vi "LabView Motor Controller.vi"() -> ()   [LabVIEW 2025]
uses:
  <vilib>/Instr/_visa.llb/VISA Configure Serial Port (Instr).vi
panel:
  in  "Start Looping Sequence":bool
  in  "Loop: Distance To Travel":dbl
  in  "Loop: Number of Cycles":dbl
  out "Current Status":string
  in  "RESET":bool
  in  "Zero":bool
  in  "Speed":dbl
  in  "Go To Location":dbl
  in  "Move Steps":dbl
  in  "VISA resource name":refnum<visa-resource-name>
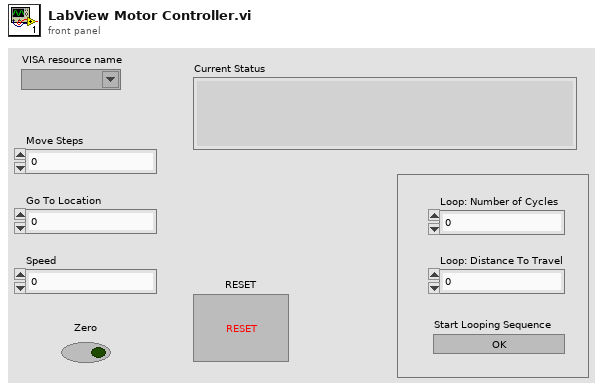
[diagram p1: front panel]
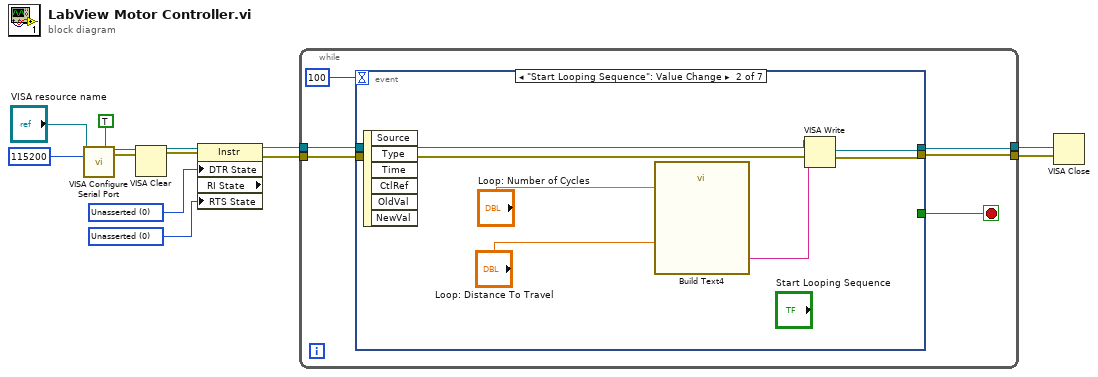
[diagram p0: block diagram]
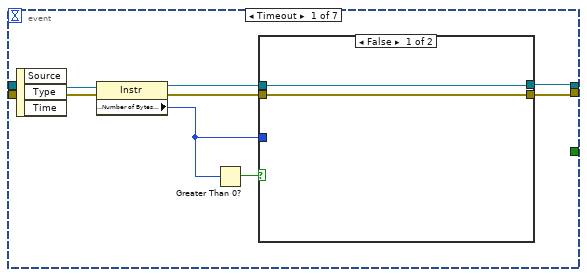
[diagram p2: hidden frame]
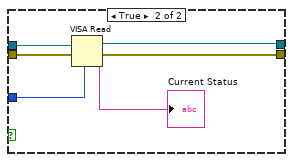
[diagram p3: hidden frame]
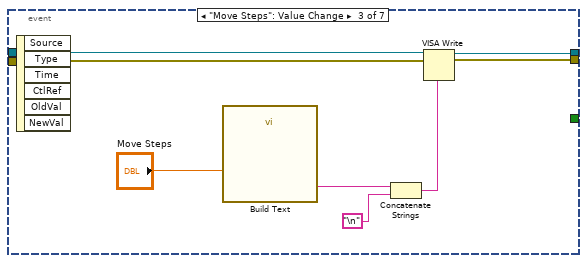
[diagram p4: hidden frame]
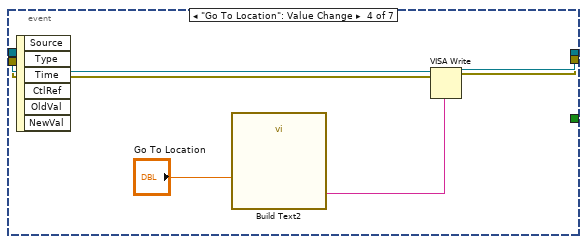
[diagram p5: hidden frame]
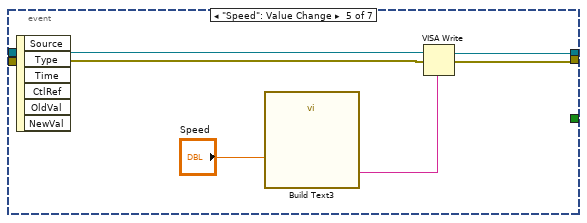
[diagram p6: hidden frame]
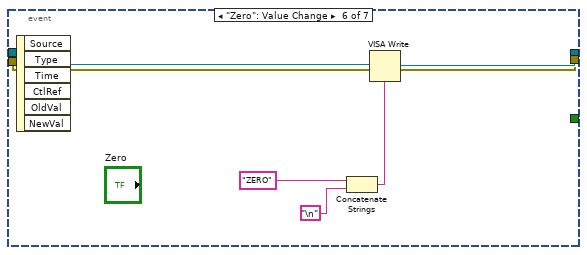
[diagram p7: hidden frame]
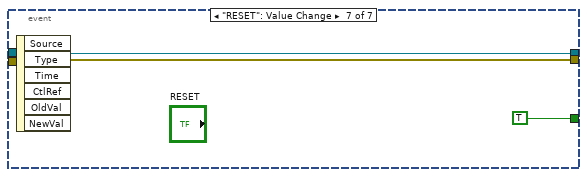
[diagram p8: hidden frame]
diagram:
  w5 = i16 0 items=["Unknown"=-1, "Unasserted"=0, "Asserted"=1] ("Serial Settings:Modem Line Settings:Line DTR State")
  w6 = i16 0 items=["Unknown"=-1, "Unasserted"=0, "Asserted"=1] ("Serial Settings:Modem Line Settings:Line RTS State")
  n1 = call-poly "VISA Configure Serial Port"("VISA resource name"="VISA resource name", "Enable Termination\nChar (T)"=TRUE ("Enable Termination\nChar (T)"), "baud rate (9600)"=u32 115200) -> ("VISA resource name out"=w4:refnum<visa-resource-name>, "error out"=w3:errorcluster)  [unwired: 11 in]
  n2 = VISA Clear(VISA resource name=w4, error in (no error)=w3) -> (VISA resource name out=w2:refnum<visa-resource-name>, error out=w1:errorcluster)
  n3 = property class="Instr" props=["DTR State", "RI State", "RTS State"](reference=w2, error in=w1, "DTR State"=w5, "RTS State"=w6) -> (reference out=w8:refnum<visa-resource-name>, error out=w7:errorcluster)  [unwired: 1 out]
  n4 = while {
    tunnel: [w17] -> w10
    tunnel: [w16] -> w9
    tunnel: w8 -> [w15]
    tunnel: w7 -> [w14]
    stop <- w19 stop-if-true
    n5 = event shown="[1] \"Start Looping Sequence\": Value Change" {
      selector: _ -> [_ _ _ _ _ _ _]
      dyn-events: _ -> [_ _ _ _ _ _ _]
      timeout: 100 -> [_ _ _ _ _ _ _]
      tunnel: w15 -> [w26 w40 w50 w55 w61 w68 w72]
      tunnel: w14 -> [w27 w39 w49 w53 w60 w69 w71]
      tunnel: [w23 w36 w47 w52 w58 w67 w72] -> w17
      tunnel: [w22 w37 w46 w51 w57 w66 w71] -> w16
      tunnel: [_ _ _ _ _ _ TRUE] -> w19
      event Timeout {
        n6 = event-data() -> ()  [unwired: 1 in, 3 out]
        n7 = property class="Instr"(reference=w26, error in=w27) -> (reference out=w25:refnum<visa-resource-name>, error out=w24:errorcluster, "Serial Settings:Number of Bytes at Serial Port"=w20:u32)
        n8 = Greater Than 0?(x=w20) -> (x > 0?=w21:bool)
        n9 = case shown="False" w21 {
          tunnel: w25 -> [w29 w35]
          tunnel: w24 -> [w28 w34]
          tunnel: [w29 w32] -> w23
          tunnel: [w28 w31] -> w22
          tunnel: w20 -> [_ w30]
          frame False {
          }
          frame True {
            n10 = VISA Read(VISA resource name=w35, byte count=w30, error in (no error)=w34) -> (VISA resource name out=w32:refnum<visa-resource-name>, read buffer=→"Current Status":string, error out=w31:errorcluster)  [unwired: 1 out]
          }
        }
      }
      event "Start Looping Sequence": Value Change {
        n11 = event-data() -> ()  [unwired: 1 in, 6 out]
        n12 = call "Build Text4"("num"="Loop: Number of Cycles", "dist"="Loop: Distance To Travel") -> ("Result"=w38:string)  [unwired: 12 in, 1 out]
        n13 = VISA Write(VISA resource name=w40, write buffer=w38, error in (no error)=w39) -> (VISA resource name out=w36:refnum<visa-resource-name>, error out=w37:errorcluster)  [unwired: 1 out]
      }
      event "Move Steps": Value Change {
        n14 = event-data() -> ()  [unwired: 1 in, 6 out]
        n15 = call "Build Text"("d"="Move Steps") -> ("Result"=w45:string)  [unwired: 13 in, 1 out]
        n16 = Concatenate Strings(w45, "\n") -> (w43:string)
        n17 = VISA Write(VISA resource name=w50, write buffer=w43, error in (no error)=w49) -> (VISA resource name out=w47:refnum<visa-resource-name>, error out=w46:errorcluster)  [unwired: 1 out]
      }
      event "Go To Location": Value Change {
        n18 = event-data() -> ()  [unwired: 1 in, 6 out]
        n19 = call "Build Text2"("d"="Go To Location") -> ("Result"=w54:string)  [unwired: 13 in, 1 out]
        n20 = VISA Write(VISA resource name=w55, write buffer=w54, error in (no error)=w53) -> (VISA resource name out=w52:refnum<visa-resource-name>, error out=w51:errorcluster)  [unwired: 1 out]
      }
      event "Speed": Value Change {
        n21 = event-data() -> ()  [unwired: 1 in, 6 out]
        n22 = call "Build Text3"("d"="Speed") -> ("Result"=w59:string)  [unwired: 13 in, 1 out]
        n23 = VISA Write(VISA resource name=w61, write buffer=w59, error in (no error)=w60) -> (VISA resource name out=w58:refnum<visa-resource-name>, error out=w57:errorcluster)  [unwired: 1 out]
      }
      event "Zero": Value Change {
        n24 = event-data() -> ()  [unwired: 1 in, 6 out]
        n25 = Concatenate Strings("ZERO", "\n") -> (w64:string)
        n26 = VISA Write(VISA resource name=w68, write buffer=w64, error in (no error)=w69) -> (VISA resource name out=w67:refnum<visa-resource-name>, error out=w66:errorcluster)  [unwired: 1 out]
      }
      event "RESET": Value Change {
        n27 = event-data() -> ()  [unwired: 1 in, 6 out]
      }
    }
  }
  n28 = VISA Close(VISA resource name=w10, error in (no error)=w9) -> ()  [unwired: 1 out]
